vi "save user data.vi"(7 "user data in":T1, 8 "error in (no error)":errorcluster, 11 "ini file":string) -> (0 "error out":errorcluster)   [LabVIEW 2024]
uses:
  <vilib>/Utility/config.llb/Write Key (String).vi
  <vilib>/Utility/config.llb/NI_LVConfig.lvlib
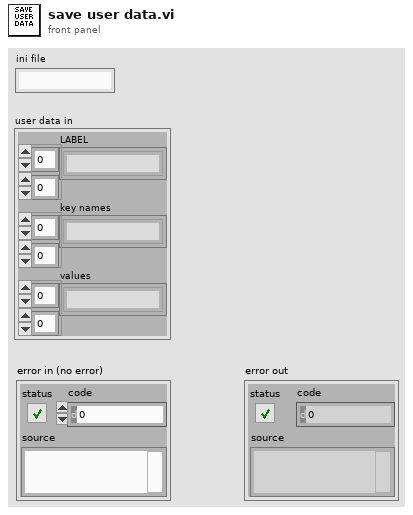
[diagram p1: front panel]
types:
  T1 = cluster{"LABEL":string[][], "key names":string[][], "values":string[][]}
  T2 = typedef "NI_LVConfig.lvlib/Config Data RefNum.ctl" = refnum<k1>
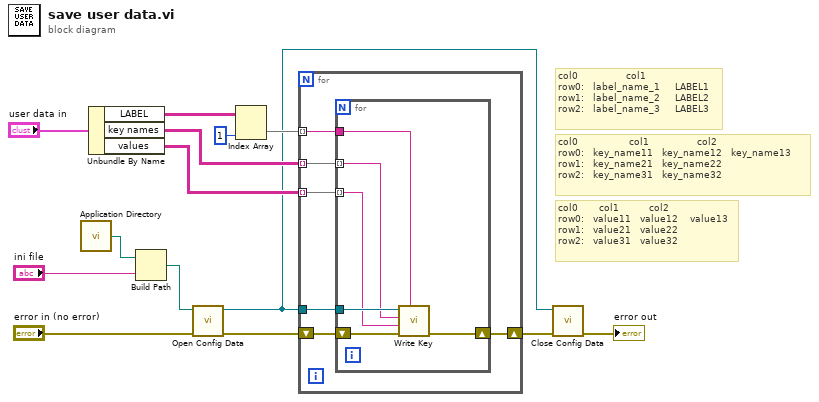
[diagram p0: block diagram]
diagram:
  # "col0       col1          col2\nrow0:   value11   value12    value13\nrow1:   value21   value22\nrow2:   value31   value32"
  # "col0                 col1                col2\nrow0:   key_name11   key_name12   key_name13\nrow1:   key_name21   key_name22 \nrow2:   key_name31   key_name32"
  # "col0                col1\nrow0:   label_name_1     LABEL1\nrow1:   label_name_2     LABEL2\nrow2:   label_name_3     LABEL3"
  n1 = call <vilib>:"Application Directory.vi"() -> ("Application Directory"=w12:path)
  n2 = Unbundle By Name("user data in") -> ("LABEL"=w8:string[][], "key names"=w5:string[][], "values"=w4:string[][])
  n3 = Build Path(base path=w12, name or relative path="ini file") -> (appended path=w13:path)
  n4 = call <vilib>:"Open Config Data.vi"("error in (no error)"="error in (no error)", "configuration file path"=w13) -> ("error out"=w9:errorcluster, "refnum"=w1:T2)  [unwired: 7 in, 1 out]
  n5 = Index Array(array=w8, index (col)=1 ("disabled index (col)")) -> (element=w6:string[])  [unwired: 1 in]
  n6 = for {
    shift-right: [w18] -> w2
    shift-left: w9 -> [w19]
    tunnel: w1 -> [w20]
    tunnel: w6 -> [w17] mode=indexing
    tunnel: w5 -> [w16] mode=indexing
    tunnel: w4 -> [w15] mode=indexing
    n7 = for {
      tunnel: w20 -> [w26]
      shift-right: [w24] -> w18
      shift-left: w19 -> [w25]
      tunnel: w17 -> [w23]
      tunnel: w16 -> [w22] mode=indexing
      tunnel: w15 -> [w21] mode=indexing
      n8 = call-poly <vilib>:"Write Key.vi"("section"=w23, "error in (no error)"=w25, "value"=w21, "key"=w22, "refnum"=w26) -> ("error out"=w24:errorcluster)  [unwired: 4 in, 2 out]
    }
  }
  n9 = call <vilib>:"Close Config Data.vi"("error in (no error)"=w2, "refnum"=w1) -> ("error out"=→"error out":errorcluster)  [unwired: 8 in, 1 out]
